vi "VsEP Read Cal Data.vi"(0 "Data Folder":path, 11 "error in (no error)":errorcluster) -> (4 "Sensitivity":dbl, 15 "error out":errorcluster)   [LabVIEW 2020]
panel:
  out "VsEP Calibration Data File":T1
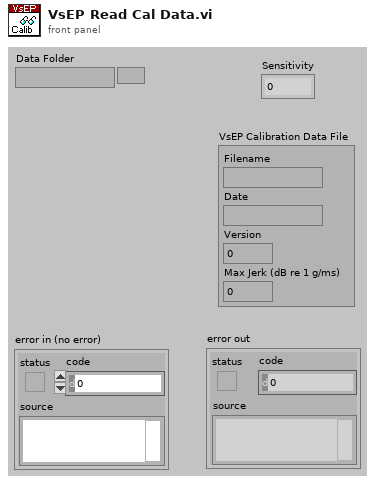
[diagram p1: front panel]
types:
  T1 = cluster{"Filename":path, "Date":string, "Version":i32, "Max Jerk (dB re 1 g/ms)":dbl}
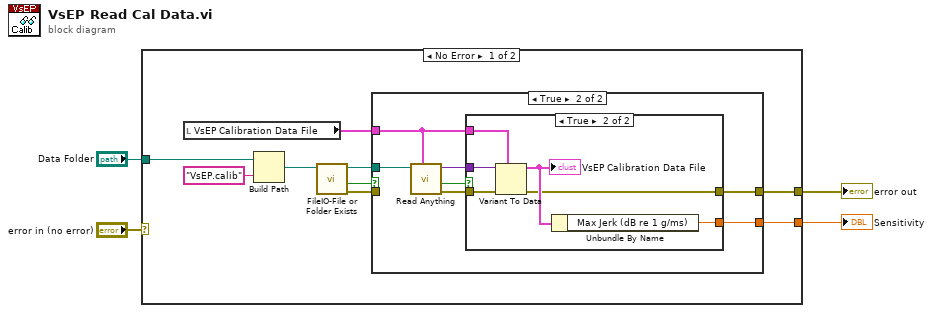
[diagram p0: block diagram]
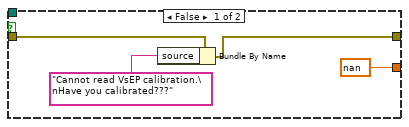
[diagram p2: hidden frame]
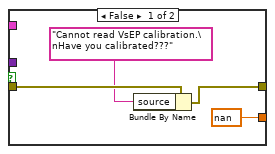
[diagram p3: hidden frame]
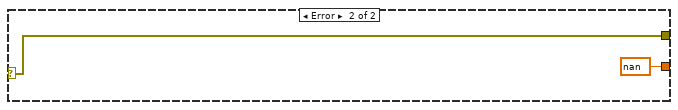
[diagram p4: hidden frame]
diagram:
  n1 = case shown="No Error" "error in (no error)" {
    selector: "error in (no error)" -> [_ w36]
    tunnel: [w5 w36] -> w4
    tunnel: [w6 nan] -> w2
    tunnel: "Data Folder" -> [w12 _]
    frame No Error {
      n2 = local read "VsEP Calibration Data File"() -> (w11:T1)
      n3 = Build Path(base path=w12, name or relative path="VsEP.calib") -> (appended path=w10:path)
      n4 = call "FileIO-File or Folder Exists.vi"("path"=w10) -> ("error out"=w7:errorcluster, "Exists?"=w8:bool, "dup path"=w9:path)  [unwired: 7 in, 1 out]
      n5 = case shown="True" w8 {
        tunnel: w11 -> [_ w20]
        tunnel: w9 -> [_ w24]
        tunnel: w7 -> [w16 _]
        tunnel: [nan w19] -> w6
        tunnel: [w14 w18] -> w5
        frame False {
          n6 = Bundle By Name(cluster=w16, "source"="Cannot read VsEP calibration.\nHave you calibrated???") -> (w14:errorcluster)
        }
        frame True {
          n7 = call "Read Anything.vi"("Type of Anything"=w20, "Path (dialog)"=w24) -> ("Error Out"=w23:errorcluster, "Found?"=w22:bool, "Anything"=w21:variant)  [unwired: 7 in]
          n8 = case shown="True" w22 {
            tunnel: w23 -> [w27 w34]
            tunnel: w21 -> [_ w33]
            tunnel: w20 -> [_ w32]
            tunnel: [nan w30] -> w19
            tunnel: [w26 w29] -> w18
            frame False {
              n9 = Bundle By Name(cluster=w27, "source"="Cannot read VsEP calibration.\nHave you calibrated???") -> (w26:errorcluster)
            }
            frame True {
              n10 = Variant To Data(error in=w34, type=w32, Variant=w33) -> (data=w31:T1, error out=w29:errorcluster)
              "VsEP Calibration Data File" <- w31
              n11 = Unbundle By Name(w31) -> ("Max Jerk (dB re 1 g/ms)"=w30:dbl)
            }
          }
        }
      }
    }
    frame Error {
    }
  }
  "error out" <- w4
  "Sensitivity" <- w2
